vi "RemoveAppender.vi"(8 "error in (no error)":errorcluster, 10 "id":string, 11 "LogManager in":refnum<class "LogManager.lvclass">) -> (0 "error out":errorcluster, 1 "found":bool, 2 "removedEnqueuer":refnum<class "Message Enqueuer.lvclass">, 3 "LogManager out":refnum<class "LogManager.lvclass">)   [LabVIEW 2026, in "Lumberjack.lvlib" / "LogManager.lvclass"]
doc: "Remove the registry entry whose id matches the input, returning the removed appender's enqueuer (so the caller can stop it) and whether a match was found. Reads then deletes against the same registry snapshot using the found index. Not-found is a benign no-op (found = FALSE, manager unchanged). Called by UnregisterAppenderMsg:Do, which posts the Snapshot (excluding the appender) before stopping it (SRS-LMBR-046)."
uses:
  LogManager.lvclass
  <vilib>/ActorFramework/Message Enqueuer/Message Enqueuer.lvclass
  LogManager.lvclass/LogManager.ctl
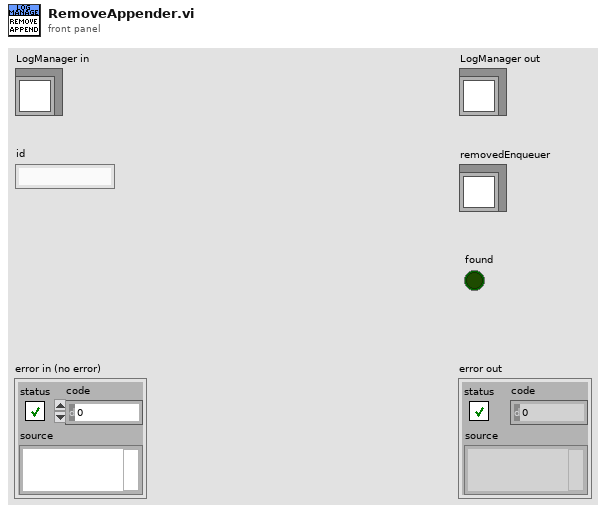
[diagram p1: front panel]
types:
  T1 = typedef "Lumberjack.lvlib/RegistryEntry.ctl" = cluster{"id":string, "enqueuer":refnum<class "Message Enqueuer.lvclass">}
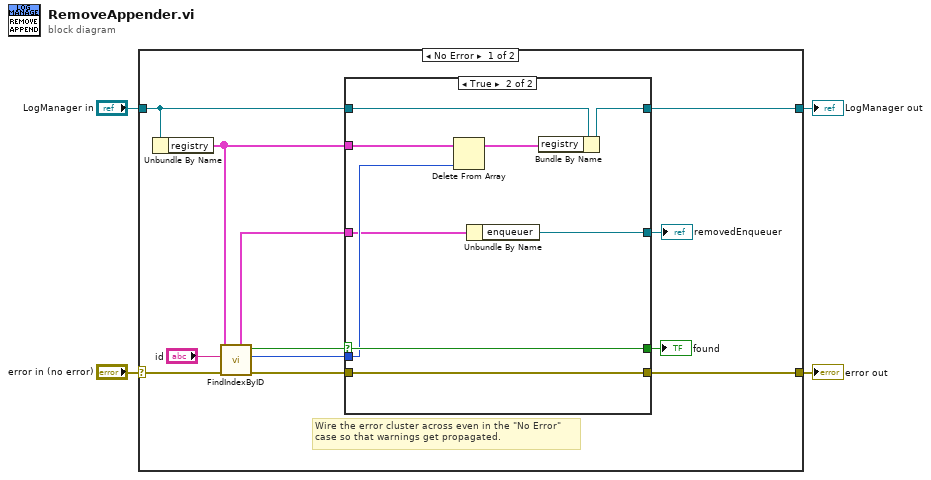
[diagram p0: block diagram]
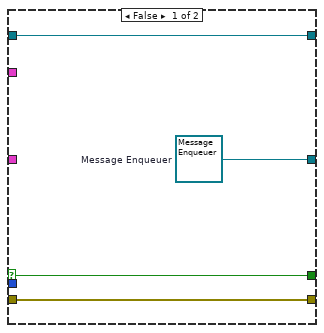
[diagram p2: hidden frame]
diagram:
  n1 = case shown="No Error" "error in (no error)" {
    selector: "error in (no error)" -> [w11 w31]
    tunnel: [w14 w31] -> w3
    tunnel: [w15 w30] -> w1
    tunnel: "LogManager in" -> [w16 w30]
    frame No Error {
      # "Wire the error cluster across even in the \"No Error\"\ncase so that warnings get propagated."
      n2 = Unbundle By Name(w16) -> ("registry"=w8:T1[])
      n3 = call "FindIndexByID.vi"("error in (no error)"=w11, "id"="id", "registry"=w8) -> ("error out"=w10:errorcluster, "index"=w6:i32, "found"=w7:bool, "registryEntry"=w5:T1)  [unwired: 5 in]
      n4 = case shown="True" w7 {
        selector: w7 -> [w18 w25]
        tunnel: w16 -> [w20 w28]
        tunnel: w10 -> [w19 w24]
        tunnel: [w20 w26] -> w15
        tunnel: [w19 w24] -> w14
        tunnel: [w18 w25] -> w13
        tunnel: [w17 w21] -> w12
        tunnel: w8 -> [_ w29]
        tunnel: w6 -> [_ w23]
        tunnel: w5 -> [_ w22]
        frame False {
          w17 = refnum<class "Message Enqueuer.lvclass"> refnum  # Message Enqueuer
        }
        frame True {
          n5 = Delete From Array(array=w29, index=w23) -> (array with subset deleted=w27:T1[])  [unwired: 1 in, 1 out]
          n6 = Unbundle By Name(w22) -> ("enqueuer"=w21:refnum<class "Message Enqueuer.lvclass">)
          n7 = Bundle By Name(cluster=w28, "registry"=w27) -> (w26:refnum<class "LogManager.lvclass">)
        }
      }
      "found" <- w13
      "removedEnqueuer" <- w12
    }
    frame Error {
    }
  }
  "error out" <- w3
  "LogManager out" <- w1
